vi "OF state PUSH.vi"(8 "errin":errorcluster, 10 "OF":string, 11 "result":string) -> (0 "error out":errorcluster)   [LabVIEW 2020]
doc: "Incremente l'état de l'OF"
uses:
  subVI/VarGLO/Global var.vi
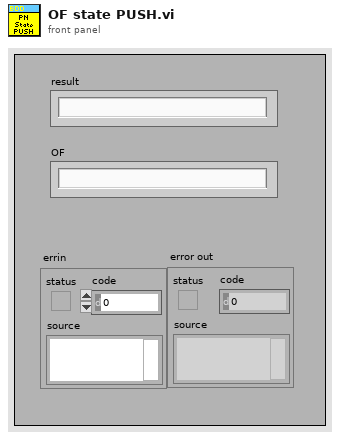
[diagram p1: front panel]
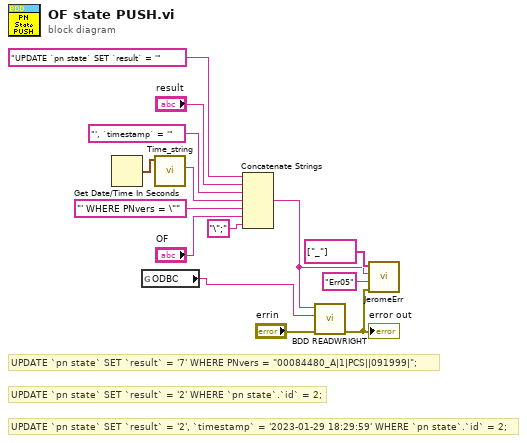
[diagram p0: block diagram]
diagram:
  # "UPDATE `pn state` SET `result` = '2', `timestamp` = '2023-01-29 18:29:59' WHERE `pn state`.`id` = 2;"
  # "UPDATE `pn state` SET `result` = '7' WHERE PNvers = \"00084480_A|1|PCS||091999|\";"
  # "UPDATE `pn state` SET `result` = '2' WHERE `pn state`.`id` = 2;"
  n1 = Get Date/Time In Seconds() -> (seconds since 1Jan1904=w9:timestamp)
  n2 = global read "Global var.vi" "ODBC"() -> (w1:string)
  n3 = call <userlib>:"Time_string.vi"("h in"=w9) -> ("heure sql"=w8:string)  [unwired: 9 in, 1 out]
  n4 = Concatenate Strings("UPDATE `pn state` SET `result` = '" ("SQL query"), "result", "', `timestamp` = '" ("chaîne"), w8, "' WHERE PNvers = \"" ("chaîne"), "OF", "\";" ("chaîne")) -> (w2:string)
  n5 = call <userlib>:"BDD READWRIGHT.vi"("errin"="errin", "DSN name"=w1, "Instruction"=w2) -> ("error out"=w3:errorcluster)  [unwired: 7 in, 1 out]
  "error out" <- w3
  n6 = call "JeromeErr.vi"("Errin"=w3, "CodeERR"="Err05", "RequetteSQL"=w2, "RetourSQL"=string[] ["_"]) -> ()  [unwired: 8 in]
